vi "Instructions Popup_VB setup.vi"(8 "error in (no error)":errorcluster) -> (0 "error out":errorcluster)   [LabVIEW 2017]
panel:
  in  "OK Button":bool
  in  "VirtualBench Device IO Control":tag
  in  "Next Button":bool
  out "String":string
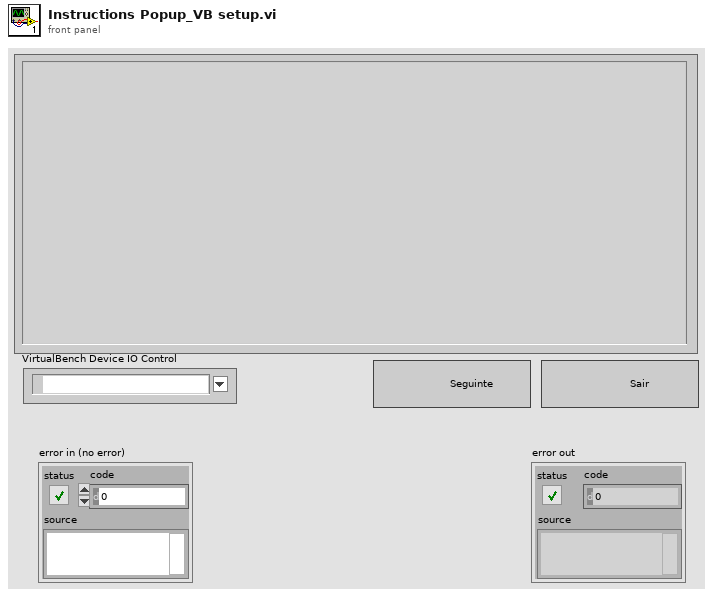
[diagram p1: front panel]
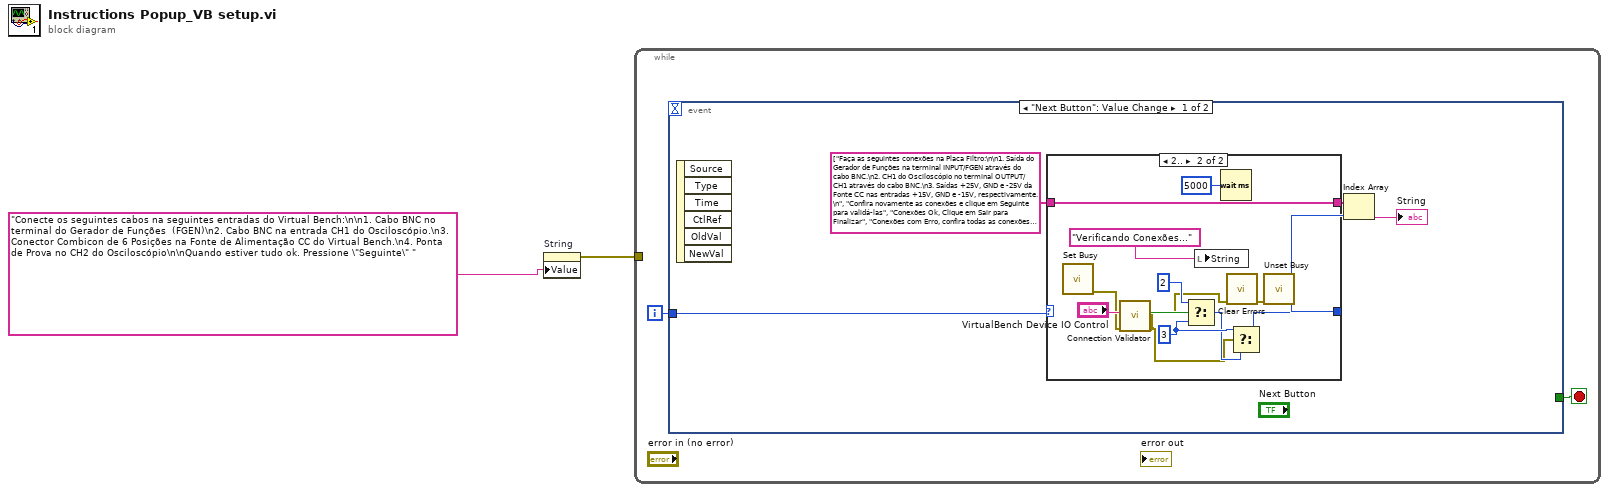
[diagram p0: block diagram]
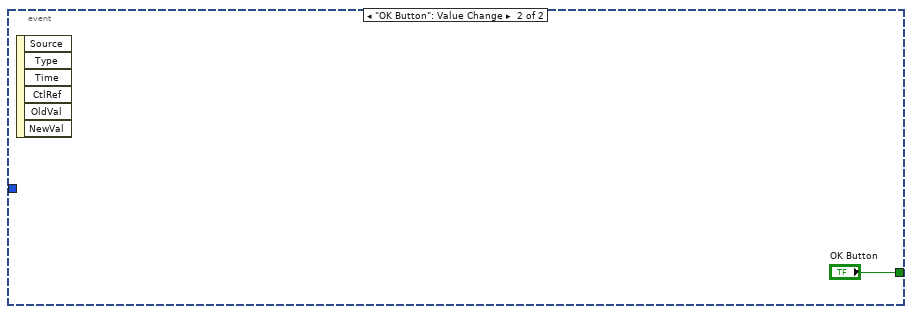
[diagram p3: hidden frame]
diagram:
  n1 = property on="String" class="Str"("Value"="Conecte os seguintes cabos na seguintes entradas do Virtual Bench:\n\n1. Cabo BNC no terminal do Gerador de Funções  (FGEN)\n2. Cabo BNC na entrada CH1 do Osciloscópio.\n3. Conector Combicon de 6 Posições na Fonte de Alimentação CC do Virtual Bench.\n4. Ponta de Prova no CH2 do Osciloscópio\n\nQuando estiver tudo ok. Pressione \"Seguinte\" ") -> (error out=w2:errorcluster)  [unwired: 2 in, 1 out]
  n2 = while {
    tunnel: w2 -> [_]
    i -> [w3]
    stop <- w4 stop-if-true
    n3 = event shown="[0] \"Next Button\": Value Change" {
      selector: _ -> [_ _]
      dyn-events: _ -> [_ _]
      timeout: _ -> [_ _]
      tunnel: [_ "OK Button"] -> w4
      tunnel: w3 -> [w5 _]
      event "Next Button": Value Change {
        n4 = event-data() -> ()  [unwired: 1 in, 6 out]
        n5 = case shown="2.." w5 {
          selector: w5 -> [w10 _]
          tunnel: [w11 w23] -> w8
          tunnel: string[] ["Faça as seguintes conexões na Placa Filtro:\n\n1. Saída do Gerador de Funções na terminal INPUT/FGEN através do cabo BNC.\n2. CH1 do Osciloscópio no terminal OUTPUT/CH1 através do cabo BNC.\n3. Saídas +25V, GND e -25V da Fonte CC nas entradas +15V, GND e -15V, respectivamente.\n", "Confira novamente as conexões e clique em Seguinte para validá-las", "Conexões Ok, Clique em Sair para Finalizar", "Conexões com Erro, confira todas as conexões e clique em OK"] ("String") -> [w11 w23]
          tunnel: [w10 w17] -> w6
          frame 0, Default {
          }
          frame 2.. {
            w16 = 3
            n6 = call <vilib>:"Set Busy.vi"() -> ("error out"=w14:errorcluster)  [unwired: 10 in, 1 out]
            n7 = call "Connection Validator.vi"("error in (no error)"=w14, "VirtualBench Device IO Control"="VirtualBench Device IO Control") -> ("error out"=w13:errorcluster, "Passed?"=w21:bool)  [unwired: 8 in]
            n8 = Select(t=2, s=w21, f=w16) -> (s? t:f=w15:i32)
            n9 = local write "String"("Verificando Conexões...") -> ()
            n10 = Wait (ms)(milliseconds to wait=u32 5000) -> ()  [unwired: 1 out]
            n11 = call <vilib>:"Clear Errors.vi"("error in (no error)"=w13) -> ("error out"=w12:errorcluster)  [unwired: 5 in, 1 out]
            n12 = Select(t=w16, s=w13, f=w15) -> (s? t:f=w17:i32)
            n13 = call <vilib>:"Unset Busy.vi"("error in (no error)"=w12) -> ()  [unwired: 10 in, 1 out]
          }
        }
        n14 = Index Array(array=w8, index=w6) -> (element=→"String":string)
      }
      event "OK Button": Value Change {
        n15 = event-data() -> ()  [unwired: 1 in, 6 out]
      }
    }
  }
